vi "GV_StartDBeditor.vi"(8 "error in (no error)":errorcluster, 11 "Gviewer in":refnum<class "Gviewer.lvclass">) -> (0 "error out":errorcluster, 3 "Gviewer out":refnum<class "Gviewer.lvclass">)   [LabVIEW 2020, in "Sgraph_lib_V1.lvlib" / "Gviewer.lvclass"]
doc: "Andre Koelewijn, 18 aug 2021\n\nStart the database editor if it was not opened already.\nBy sending the request to the Gserver if the DBeditor was already started,\nthe actual starting of the DB editor will occur on the reply of the Gserver.\nWhen the DBeditor was not started, this wil open the DBeditor application dynamically."
uses:
  Gviewer.lvclass
  Gserver/controls/Typedef_QueryType.ctl
  Gserver/Gserver.lvclass
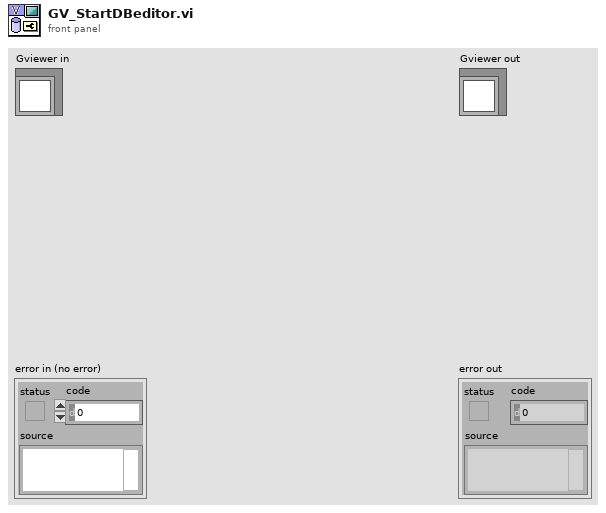
[diagram p1: front panel]
types:
  T1 = typedef "Sgraph_lib_V1.lvlib/Gserver.lvclass/Typedef_QueryType.ctl" = enum16{"Subscribe", "DataRequest", "RequestAllTags", "RequestIniPath", "FAMMstarted", "SetClientOptions", "GviewerUpdate", "OpenNewGraph", "CloseClient", "CloseAllClients", "Close Gserver", "OpenMemoryMap", "MeMapDataRequest", "MeMapDataResponse", "OpenDBeditor", "CheckDBeditorRunning", "StoppedDBeditor", "SaveDB_TAGpropRecord", "ConfirmDB_TAGpropSave"}
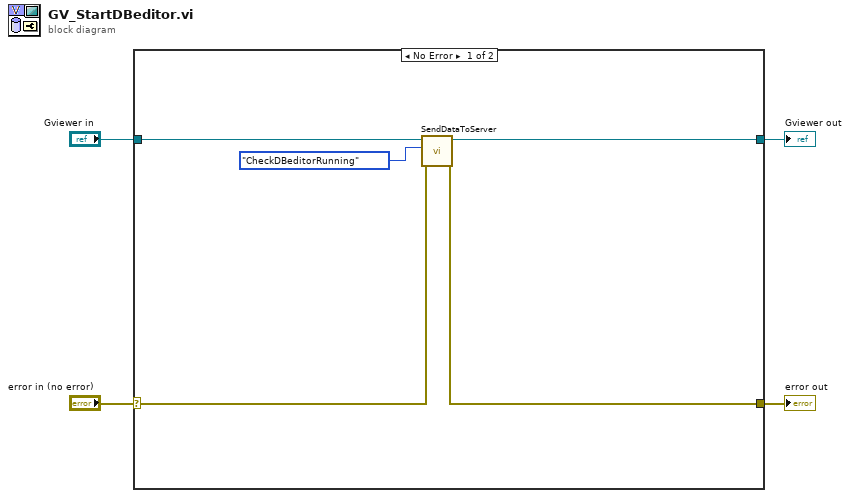
[diagram p0: block diagram]
diagram:
  n1 = case shown="No Error" "error in (no error)" {
    selector: "error in (no error)" -> [w6 w11]
    tunnel: [w5 w11] -> w3
    tunnel: [w8 w10] -> w1
    tunnel: "Gviewer in" -> [w7 w10]
    frame No Error {
      n2 = call "SendDataToServer.vi"("error in (no error)"=w6, "Query_type"=Typedef_QueryType."CheckDBeditorRunning", "Gviewer in"=w7) -> ("error out"=w5:errorcluster, "Gviewer out"=w8:refnum<class "Gviewer.lvclass">)  [unwired: 7 in]
    }
    frame Error {
    }
  }
  "error out" <- w3
  "Gviewer out" <- w1
